vi "Create Resource Instance.vi"(10 "instance":u8, 11 "niUSRP Rx DSP v2 FPGA in":refnum<class "niUSRP Rx DSP v2 FPGA.lvclass">) -> (0 "RxDspSupport":u64, 2 "address space collection":refnum<class "Address Space Collection.lvclass">, 3 "niUSRP Rx DSP v2 FPGA out":refnum<class "niUSRP Rx DSP v2 FPGA.lvclass">)   [LabVIEW 2025, in "niUSRP Rx DSP v2 FPGA.lvclass"]
uses:
  niUSRP Rx DSP v2 FPGA.lvclass
  <instrlib>/_niInstr/Instruction Framework/v1/FPGA/Interfaces/Address Space Collection/Address Space Collection.lvclass
  <instrlib>/_niInstr/DSP Control/Common/v2/FPGA/Resampling/Harness Type.ctl
  <instrlib>/_niInstr/DSP Control/Common/v2/FPGA/Equalization/Registers/Equalization Filter Type.ctl
  <instrlib>/_niInstr/Instruction Framework/v1/FPGA/Collection Builder/Collection Builder.lvclass
  <instrlib>/_niInstr/DSP Control/Interface/v1/FPGA/niInstr DSP Control Interface v1 FPGA.lvlib
  <instrlib>/_niInstr/Basic Elements/v1/FPGA/niInstr Basic Elements v1 FPGA.lvlib
  <instrlib>/_niInstr/DSP Control/Common/v2/FPGA/Equalization/Registers/Equalization Registers.lvclass
  <instrlib>/_niInstr/DSP Control/Common/v2/FPGA/Resampling/Resampler Harness.lvclass
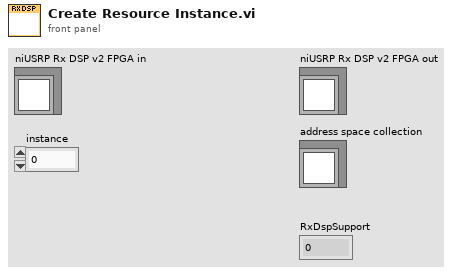
[diagram p1: front panel]
types:
  T1 = typedef "niInstr DSP Control Common v2 FPGA.lvlib/Equalization Registers.lvclass/Equalization Filter Type.ctl" = enum8{"Undefined", "Single", "Complex", "Matrix"}
  T2 = typedef "niInstr DSP Control Common v2 FPGA.lvlib/Resampler Harness.lvclass/Harness Type.ctl" = enum16{"None", "Integer Linear", "Integer List", "Integer-Exponential", "Fixed Rational", "Fractional (16-bit Delay)", "Fractional (18-bit Delay)", "Rational List", "External", "External and Fractional"}
  T3 = typedef "niInstr Address Space Collection Builder v1 FPGA.lvlib/Parent Metadata.ctl" = cluster{"UID":u16, "version":u16, "oldest compatible version":u16}
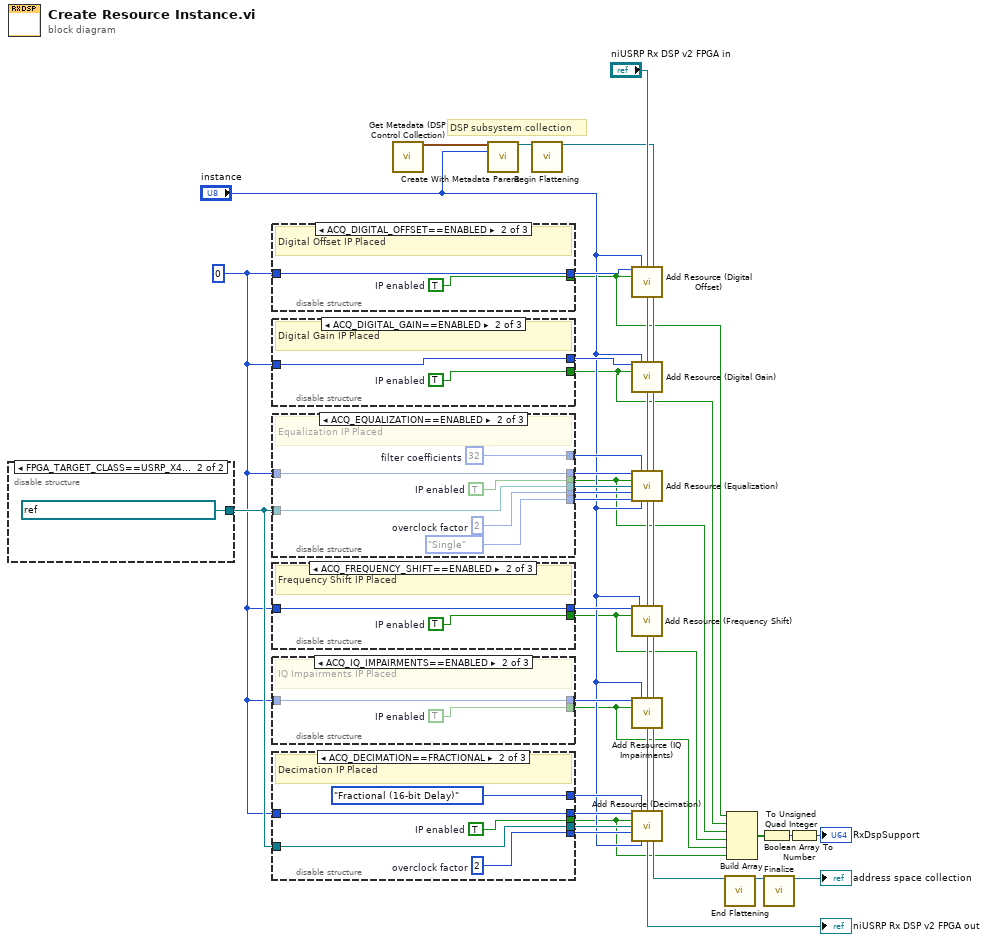
[diagram p0: block diagram]
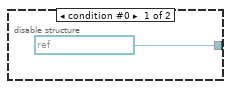
[diagram p2: hidden frame]
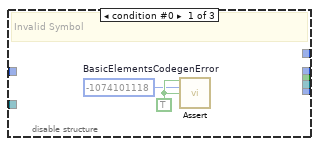
[diagram p3: hidden frame]
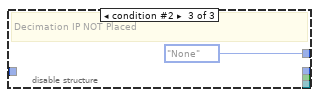
[diagram p4: hidden frame]
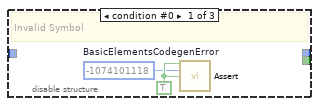
[diagram p5: hidden frame]
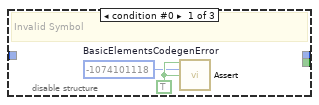
[diagram p7: hidden frame]
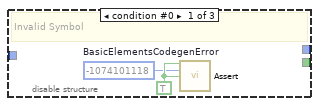
[diagram p9: hidden frame]
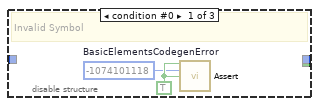
[diagram p11: hidden frame]
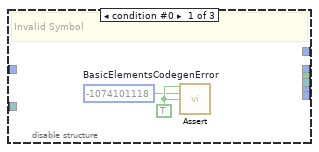
[diagram p13: hidden frame]
diagram:
  w14 = u8 0 ("instance")
  # "DSP subsystem collection"
  n1 = disable-structure shown="FPGA_TARGET_CLASS==USRP_X410||FPGA_TARGET_CLASS==USRP_X410__EMBEDDED____UNSUPPORTED" {
    disable-tunnel: [refnum<k21> "Data Clock x2" ("clock x2") refnum<k21> "Daughterboard 0\\Data Clock x2" ("clock x2")] -> w41
    frame condition #0 {
    }
    frame condition #1 (active) {
    }
  }
  n2 = disable-structure shown="ACQ_DIGITAL_OFFSET==ENABLED" {
    disable-tunnel: [_ w49 _] -> w8
    disable-tunnel: [_ w48 _] -> w43
    disable-tunnel: w14 -> [_ w48 _]
    frame condition #0 {
      w47 = TRUE ("assert")
      w46 = -1074101118  # BasicElementsCodegenError
      # "Invalid Symbol"
      n3 = call <instrlib>:"Assert.vi"("assert"=w47, "error code"=w46, "enable show error"=w47) -> ()  [unwired: 13 in]
    }
    frame condition #1 (active) {
      w49 = TRUE  # IP enabled
      # "Digital Offset IP Placed"
    }
    frame condition #2 {
      # "Digital Offset IP NOT Placed"
    }
  }
  n4 = disable-structure shown="ACQ_DIGITAL_GAIN==ENABLED" {
    disable-tunnel: [_ w52 _] -> w18
    disable-tunnel: [_ w53 _] -> w7
    disable-tunnel: w14 -> [_ w52 _]
    frame condition #0 {
      w51 = TRUE ("assert")
      w50 = -1074101118  # BasicElementsCodegenError
      # "Invalid Symbol"
      n5 = call <instrlib>:"Assert.vi"("assert"=w51, "error code"=w50, "enable show error"=w51) -> ()  [unwired: 13 in]
    }
    frame condition #1 (active) {
      w53 = TRUE  # IP enabled
      # "Digital Gain IP Placed"
    }
    frame condition #2 {
      # "Digital Gain IP NOT Placed"
    }
  }
  n6 = disable-structure shown="ACQ_EQUALIZATION==ENABLED" {
    disable-tunnel: [_ w56 _] -> w16
    disable-tunnel: [_ w61 _] -> w6
    disable-tunnel: [_ w60 _] -> w15
    disable-tunnel: [_ w57 _] -> w42
    disable-tunnel: [_ w59 _] -> w17
    disable-tunnel: [_ Equalization_Filter_Type."Single" ("filter type") _] -> w40
    disable-tunnel: w41 -> [_ w57 _]
    disable-tunnel: w14 -> [_ w56 _]
    frame condition #0 {
      w55 = TRUE ("assert")
      w54 = -1074101118  # BasicElementsCodegenError
      # "Invalid Symbol"
      n7 = call <instrlib>:"Assert.vi"("assert"=w55, "error code"=w54, "enable show error"=w55) -> ()  [unwired: 13 in]
    }
    frame condition #1 {
      w59 = u8 32  # filter coefficients
      w60 = u8 2  # overclock factor
      w61 = TRUE  # IP enabled
      # "Equalization IP Placed"
    }
    frame condition #2 (active) {
      # "Equalization IP NOT Placed"
    }
  }
  n8 = disable-structure shown="ACQ_FREQUENCY_SHIFT==ENABLED" {
    disable-tunnel: [_ w64 _] -> w19
    disable-tunnel: [_ w65 _] -> w5
    disable-tunnel: w14 -> [_ w64 _]
    frame condition #0 {
      w63 = TRUE ("assert")
      w62 = -1074101118  # BasicElementsCodegenError
      # "Invalid Symbol"
      n9 = call <instrlib>:"Assert.vi"("assert"=w63, "error code"=w62, "enable show error"=w63) -> ()  [unwired: 13 in]
    }
    frame condition #1 (active) {
      w65 = TRUE  # IP enabled
      # "Frequency Shift IP Placed"
    }
    frame condition #2 {
      # "Frequency Shift IP NOT Placed"
    }
  }
  n10 = disable-structure shown="ACQ_IQ_IMPAIRMENTS==ENABLED" {
    disable-tunnel: [_ w68 _] -> w20
    disable-tunnel: [_ w69 _] -> w4
    disable-tunnel: w14 -> [_ w68 _]
    frame condition #0 {
      w67 = TRUE ("assert")
      w66 = -1074101118  # BasicElementsCodegenError
      # "Invalid Symbol"
      n11 = call <instrlib>:"Assert.vi"("assert"=w67, "error code"=w66, "enable show error"=w67) -> ()  [unwired: 13 in]
    }
    frame condition #1 {
      w69 = TRUE  # IP enabled
      # "IQ Impairments IP Placed"
    }
    frame condition #2 (active) {
      # "IQ Impairments IP NOT Placed"
    }
  }
  n12 = disable-structure shown="ACQ_DECIMATION==FRACTIONAL" {
    disable-tunnel: [_ w72 _] -> w22
    disable-tunnel: [_ w76 _] -> w3
    disable-tunnel: [_ w75 _] -> w24
    disable-tunnel: [_ w73 _] -> w23
    disable-tunnel: [_ Harness_Type."Fractional (16-bit Delay)" ("harness type") Harness_Type."None" ("harness type")] -> w21
    disable-tunnel: w41 -> [_ w73 _]
    disable-tunnel: w14 -> [_ w72 _]
    frame condition #0 {
      w71 = TRUE ("assert")
      w70 = -1074101118  # BasicElementsCodegenError
      # "Invalid Symbol"
      n13 = call <instrlib>:"Assert.vi"("assert"=w71, "error code"=w70, "enable show error"=w71) -> ()  [unwired: 13 in]
    }
    frame condition #1 (active) {
      w75 = u8 2  # overclock factor
      w76 = TRUE  # IP enabled
      # "Decimation IP Placed"
    }
    frame condition #2 {
      # "Decimation IP NOT Placed"
    }
  }
  n14 = call <instrlib>:"Get Metadata (DSP Control Collection).vi"() -> ("parent metadata"=w37:T3)  [unwired: 15 in]
  n15 = call <instrlib>:"Create With Metadata Parent.vi"("parent metadata"=w37, "instance (0)"="instance") -> ("collection builder"=w35:refnum<class "Collection Builder.lvclass">)  [unwired: 13 in]
  n16 = call <instrlib>:"Begin Flattening.vi"("collection builder in"=w35) -> ("collection builder out"=w36:refnum<class "Collection Builder.lvclass">)  [unwired: 14 in]
  n17 = call-dynamic "Add Resource (Digital Offset).vi"("instance"=w43, "channel"="instance", "acq in"="niUSRP Rx DSP v2 FPGA in", "collection builder in"=w36, "IP enabled"=w8) -> ("acq out"=w25:refnum<class "niUSRP Rx DSP v2 FPGA.lvclass">, "collection builder out"=w28:refnum<class "Collection Builder.lvclass">)  [unwired: 9 in]
  n18 = call-dynamic "Add Resource (Digital Gain).vi"("instance"=w18, "channel"="instance", "acq in"=w25, "collection builder in"=w28, "IP enabled"=w7) -> ("acq out"=w26:refnum<class "niUSRP Rx DSP v2 FPGA.lvclass">, "collection builder out"=w27:refnum<class "Collection Builder.lvclass">)  [unwired: 9 in]
  n19 = call-dynamic "Add Resource (Equalization).vi"("instance"=w16, "number of filter coefficients"=w17, "acq in"=w26, "collection builder in"=w27, "IP enabled"=w6, "overclock"=w42, "overclock factor"=w15, "filter type"=w40, "channel"="instance") -> ("acq out"=w29:refnum<class "niUSRP Rx DSP v2 FPGA.lvclass">, "collection builder out"=w30:refnum<class "Collection Builder.lvclass">)  [unwired: 5 in]
  n20 = call-dynamic "Add Resource (Frequency Shift).vi"("instance"=w19, "channel"="instance", "acq in"=w29, "collection builder in"=w30, "IP enabled"=w5) -> ("acq out"=w31:refnum<class "niUSRP Rx DSP v2 FPGA.lvclass">, "collection builder out"=w32:refnum<class "Collection Builder.lvclass">)  [unwired: 9 in]
  n21 = call-dynamic "Add Resource (IQ Impairments).vi"("instance"=w20, "channel"="instance", "acq in"=w31, "collection builder in"=w32, "IP enabled"=w4) -> ("acq out"=w33:refnum<class "niUSRP Rx DSP v2 FPGA.lvclass">, "collection builder out"=w34:refnum<class "Collection Builder.lvclass">)  [unwired: 9 in]
  n22 = call-dynamic "Add Resource (Decimation).vi"("instance"=w22, "harness type"=w21, "acq in"=w33, "collection builder in"=w34, "IP enabled"=w3, "overclock"=w23, "overclock factor"=w24, "channel"="instance") -> ("acq out"=→"niUSRP Rx DSP v2 FPGA out":refnum<class "niUSRP Rx DSP v2 FPGA.lvclass">, "collection builder out"=w12:refnum<class "Collection Builder.lvclass">)  [unwired: 6 in]
  n23 = call <instrlib>:"End Flattening.vi"("collection builder in"=w12) -> ("collection builder out"=w13:refnum<class "Collection Builder.lvclass">)  [unwired: 14 in]
  n24 = Build Array(w8, w7, w6, w5, w4, w3) -> (w9:bool[])
  n25 = Boolean Array To Number(Boolean array=w9) -> (number=w2:u8)
  n26 = call <instrlib>:"Finalize.vi"("collection builder in"=w13) -> ("address space collection"=→"address space collection":refnum<class "Address Space Collection.lvclass">)  [unwired: 14 in]
  n27 = To Unsigned Quad Integer(1:w2) -> (0:→"RxDspSupport":u64)
